vi "TurnCalculator.vi"(0 "Desired Angle":dbl=0.026 format="%#_13g", 1 "Loading Tool":u16(ring) items=["Metric", "English"], 2 "Measured Coordinates (mm)":dbl[](array[numeric]), 3 "Top Left Corner Desired Coordinates (mm)":dbl[](array[numeric]), 4 "Y Side length (m)":dbl=0.09643 format="%#_13g", 5 "X Side length (m)":dbl=0.095426 format="%#_13g") -> (6 "Angle Knob Rotations":dbl, 7 "X Knob Rotations":dbl, 8 "Y Knob Rotations":dbl)   [LabVIEW 2016]
uses:
  <vilib>/Analysis/baseanly.llb/Mean (DBL).vi
  <vilib>/Analysis/NI_AALBase.lvlib
panel:
  out "Y displacement (microns)":dbl
  out "X displacement (microns)":dbl
  out "Radians from Ideal":dbl format="%0.5f"
  out "Degrees per Rotation Angle":dbl=1.0 format="%#_13g"
  out "Microns per Rotation Y":dbl=1.0 format="%#_13g"
  out "Microns per Rotation X":dbl=1.0 format="%#_13g"
  # "Inputs"
  # "Outputs"
  # "Tool Information"
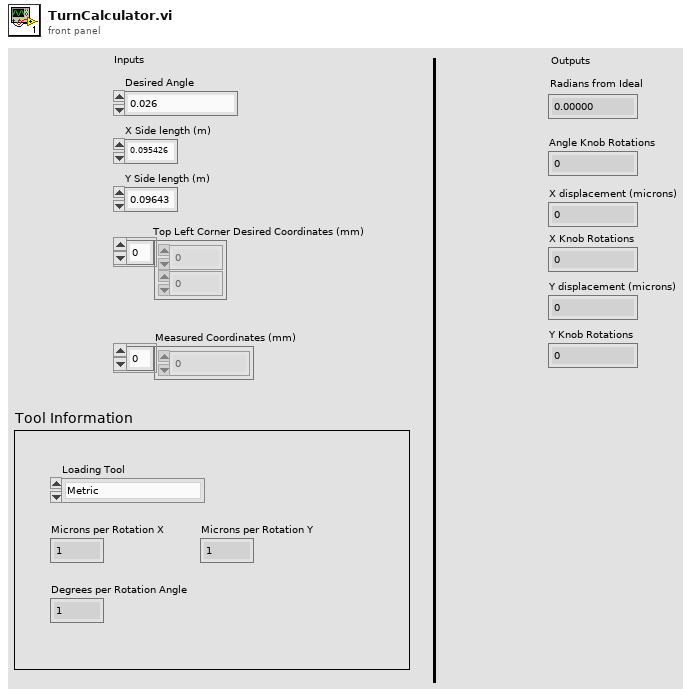
[diagram p1: front panel]
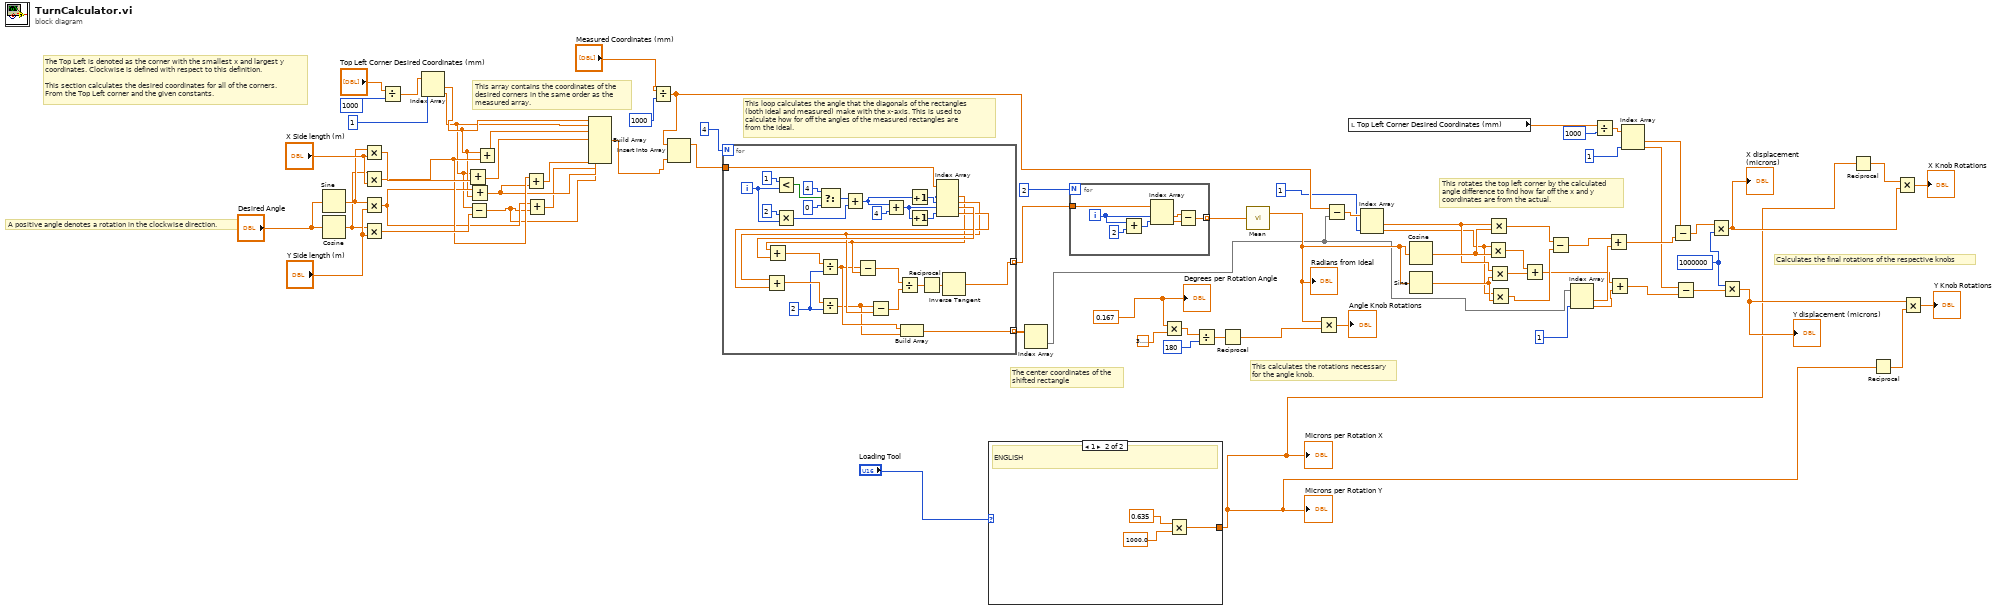
[diagram p0: block diagram]
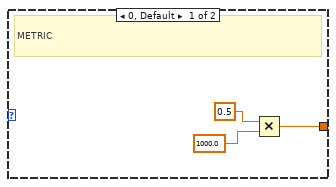
[diagram p2: hidden frame]
diagram:
  w1 = 0.167
  w20 = 1000000
  # "Calculates the final rotations of the respective knobs"
  # "This rotates the top left corner by the calculated\nangle difference to find how far off the x and y \ncoordinates are from the actual."
  # "This calculates the rotations necessary\nfor the angle knob."
  # "The center coordinates of the\nshifted rectangle"
  # "This loop calculates the angle that the diagonals of the rectangles\n(both ideal and measured) make with the x-axis. This is used to\ncalculate how for off the angles of the measured rectangles are\nfrom the ideal."
  # "This array contains the coordinates of the\ndesired corners in the same order as the\nmeasured array."
  # "The Top Left is denoted as the corner with the smallest x and largest y\ncoordinates. Clockwise is defined with respect to this definition.\n\nThis section calculates the desired coordinates for all of the corners.\nFrom the Top Left corner and the given constants."
  # "A positive angle denotes a rotation in the clockwise direction."
  n1 = Sine(x="Desired Angle") -> (sin(x)=w7:dbl)
  n2 = Cosine(x="Desired Angle") -> (cos(x)=w6:dbl)
  n3 = Multiply(x=w7, y="X Side length (m)") -> (x*y=w69:dbl)
  n4 = Multiply(x=w6, y="X Side length (m)") -> (x*y=w68:dbl)
  n5 = Multiply(x=w7, y="Y Side length (m)") -> (x*y=w67:dbl)
  n6 = Multiply(x=w6, y="Y Side length (m)") -> (x*y=w70:dbl)
  n7 = Divide(x="Top Left Corner Desired Coordinates (mm)", y=1000) -> (x/y=w61:dbl[])
  n8 = Index Array(array=w61, index #2=1 ("index")) -> (element #1=w9:dbl, element #2=w5:dbl)  [unwired: 1 in]
  n9 = Add(x=w5, y=w69) -> (x+y=w71:dbl)
  n10 = Subtract(x=w5, y=w70) -> (x-y=w56:dbl)
  n11 = Add(x=w67, y=w9) -> (x+y=w65:dbl)
  n12 = Add(x=w9, y=w68) -> (x+y=w72:dbl)
  n13 = Add(x=w68, y=w65) -> (x+y=w55:dbl)
  n14 = Add(x=w67, y=w56) -> (x+y=w54:dbl)
  n15 = Build Array(w9, w5, w72, w71, w55, w54, w65, w56) -> (w64:dbl[])
  n16 = Divide(x="Measured Coordinates (mm)", y=1000) -> (x/y=w44:dbl[])
  n17 = Insert Into Array(array=w44, new element=w64) -> (w63:dbl[])  [unwired: 1 in]
  n18 = for {
    N: 4 -> [_]
    tunnel: w63 -> [w103]
    tunnel: [w78] -> w58 mode=indexing
    tunnel: [w75] -> w45 mode=indexing
    i -> [w94]
    w86 = 2
    n19 = Less?(x=1, y=w94) -> (x < y?=w92:bool)
    n20 = Multiply(x=2, y=w94) -> (x*y=w91:i32)
    n21 = Select(t=4, s=w92, f=0) -> (s? t:f=w96:i32)
    n22 = Add(x=w96, y=w91) -> (x+y=w79:i32)
    n23 = Add(x=w79, y=4) -> (x+y=w101:i32)
    n24 = Increment(x=w79) -> (x+1=w100:i32)
    n25 = Increment(x=w101) -> (x+1=w102:i32)
    n26 = Index Array(array=w103, index #1=w79, index #2=w100, index #3=w101, index #4=w102) -> (element #1=w80:dbl, element #2=w85:dbl, element #3=w90:dbl, element #4=w89:dbl)
    n27 = Add(x=w85, y=w89) -> (x+y=w88:dbl)
    n28 = Add(x=w80, y=w90) -> (x+y=w87:dbl)
    n29 = Divide(x=w87, y=w86) -> (x/y=w77:dbl)
    n30 = Divide(x=w88, y=w86) -> (x/y=w76:dbl)
    n31 = Subtract(x=w77, y=w80) -> (x-y=w83:dbl)
    n32 = Subtract(x=w76, y=w85) -> (x-y=w84:dbl)
    n33 = Divide(x=w83, y=w84) -> (x/y=w82:dbl)
    n34 = Build Array(w77, w76) -> (w75:dbl[])
    n35 = Reciprocal(x=w82) -> (1/x=w81:dbl)
    n36 = Inverse Tangent(1:w81) -> (0:w78:dbl)
  }
  n37 = case shown="1" "Loading Tool" {
    tunnel: [w104 w107] -> w2
    frame 0, Default {
      # "METRIC"
      n38 = Multiply(x=0.5, y=1000.0) -> (x*y=w104:dbl)
    }
    frame 1 {
      # "ENGLISH"
      n39 = Multiply(x=0.635, y=1000.0) -> (x*y=w107:dbl)
    }
  }
  "Microns per Rotation X" <- w2
  "Microns per Rotation Y" <- w2
  n40 = Index Array(array=w45) -> (element=w31:dbl[])  [unwired: 2 in]
  n41 = for {
    N: 2 -> [_]
    tunnel: w58 -> [w116]
    tunnel: [w110] -> w53 mode=indexing
    i -> [w114]
    n42 = Add(x=w114, y=2) -> (x+y=w115:i32)
    n43 = Index Array(array=w116, index #1=w114, index #2=w115) -> (element #1=w112:dbl, element #2=w111:dbl)
    n44 = Subtract(x=w112, y=w111) -> (x-y=w110:dbl)
  }
  n45 = Multiply(x=w1, y=3.141592653589793) -> (x*y=w50:dbl)
  n46 = Divide(x=w50, y=180) -> (x/y=w48:dbl)
  n47 = Reciprocal(x=w48) -> (1/x=w47:dbl)
  n48 = call-poly <vilib>:"Mean.vi"("X"=w53) -> ("mean"=w41:dbl)  [unwired: 1 out]
  "Radians from Ideal" <- w41
  n49 = Multiply(x=w41, y=w47) -> (x*y=→"Angle Knob Rotations":dbl)
  n50 = Subtract(x=w44, y=w31) -> (x-y=w43:dbl[])
  n51 = local read "Top Left Corner Desired Coordinates (mm)"() -> (w12:dbl[])
  n52 = Index Array(array=w43, index #2=1) -> (element #1=w38:dbl, element #2=w37:dbl)  [unwired: 1 in]
  n53 = Cosine(x=w41) -> (cos(x)=w40:dbl)
  n54 = Sine(x=w41) -> (sin(x)=w39:dbl)
  n55 = Multiply(x=w37, y=w40) -> (x*y=w35:dbl)
  n56 = Multiply(x=w38, y=w40) -> (x*y=w33:dbl)
  n57 = Multiply(x=w38, y=w39) -> (x*y=w36:dbl)
  n58 = Multiply(x=w37, y=w39) -> (x*y=w34:dbl)
  n59 = Add(x=w35, y=w36) -> (x+y=w27:dbl)
  n60 = Subtract(x=w33, y=w34) -> (x-y=w28:dbl)
  n61 = Index Array(array=w31, index #2=1) -> (element #1=w29:dbl, element #2=w26:dbl)  [unwired: 1 in]
  n62 = Divide(x=w12, y=1000) -> (x/y=w10:dbl[])
  n63 = Add(x=w28, y=w29) -> (x+y=w24:dbl)
  n64 = Add(x=w27, y=w26) -> (x+y=w22:dbl)
  n65 = Index Array(array=w10, index #2=1) -> (element #1=w25:dbl, element #2=w23:dbl)  [unwired: 1 in]
  n66 = Subtract(x=w25, y=w24) -> (x-y=w21:dbl)
  n67 = Subtract(x=w23, y=w22) -> (x-y=w19:dbl)
  n68 = Multiply(x=w21, y=w20) -> (x*y=w15:dbl)
  "X displacement (microns)" <- w15
  n69 = Multiply(x=w20, y=w19) -> (x*y=w17:dbl)
  "Y displacement (microns)" <- w17
  n70 = Reciprocal(x=w2) -> (1/x=w16:dbl)
  n71 = Reciprocal(x=w2) -> (1/x=w18:dbl)
  n72 = Multiply(x=w16, y=w15) -> (x*y=→"X Knob Rotations":dbl)
  n73 = Multiply(x=w17, y=w18) -> (x*y=→"Y Knob Rotations":dbl)
  "Degrees per Rotation Angle" <- w1
